vi "Open Excel.vi"(8 "error in (no error)":errorcluster, 9 "Visible":bool, 11 "Excel Interface in":refnum<class "Excel Interface.lvclass">) -> (0 "error out":errorcluster, 3 "Excel Interface out":refnum<class "Excel Interface.lvclass">)   [LabVIEW 2013, in "Excel Interface.lvclass"]
uses:
  Excel Interface.lvclass
  Excel Interface.lvclass/Excel Interface.ctl
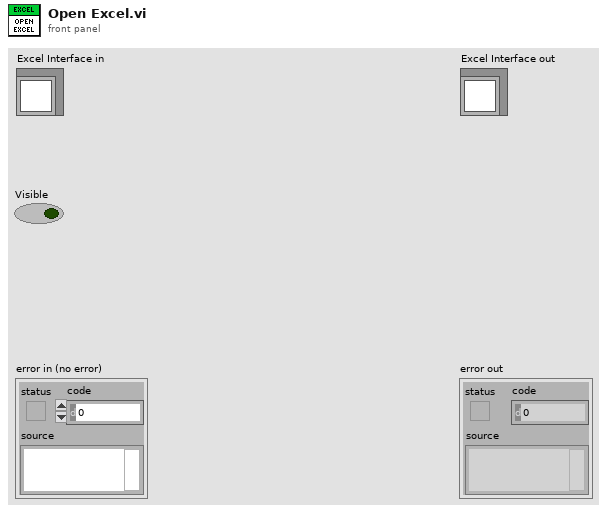
[diagram p1: front panel]
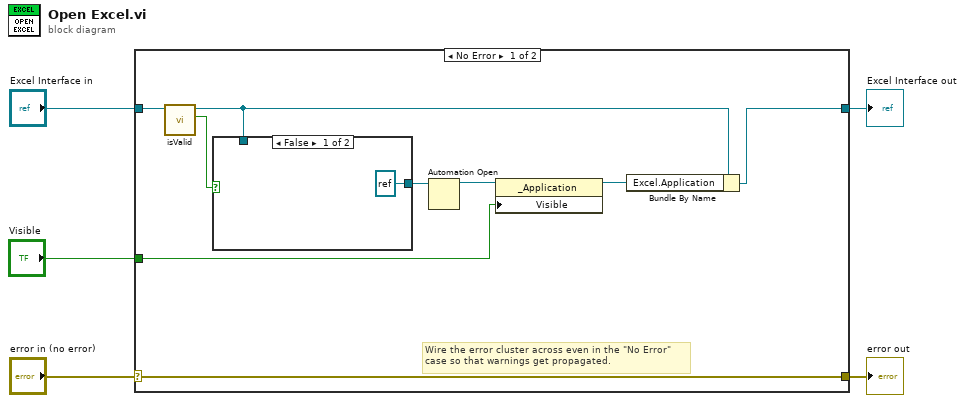
[diagram p0: block diagram]
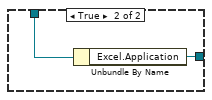
[diagram p2: hidden frame]
diagram:
  n1 = case shown="No Error" "error in (no error)" {
    selector: "error in (no error)" -> [w14 w19]
    tunnel: [w14 w19] -> w4
    tunnel: [w11 w18] -> w2
    tunnel: "Excel Interface in" -> [w9 w18]
    tunnel: "Visible" -> [w12 _]
    frame No Error {
      # "Wire the error cluster across even in the \"No Error\"\ncase so that warnings get propagated."
      n2 = call-dynamic "isValid.vi"("Excel Interface in"=w9) -> ("valid"=w7:bool, "Excel Interface out"=w8:refnum<class "Excel Interface.lvclass">)  [unwired: 8 in, 1 out]
      n3 = case shown="False" w7 {
        tunnel: w8 -> [_ w17]
        tunnel: [refnum<k7> refnum ("Excel.Application") w16] -> w6
        frame False {
        }
        frame True {
          n4 = Unbundle By Name(w17) -> ("Excel.Application"=w16:refnum<k7>)
        }
      }
      n5 = Automation Open(Automation Refnum=w6) -> (Automation Refnum=w13:refnum<k7>)  [unwired: 3 in, 1 out]
      n6 = property class="_Application"(reference=w13, "Visible"=w12) -> (reference out=w10:refnum<k7>)  [unwired: 1 in, 1 out]
      n7 = Bundle By Name(cluster=w8, "Excel.Application"=w10) -> (w11:refnum<class "Excel Interface.lvclass">)
    }
    frame Error {
    }
  }
  "error out" <- w4
  "Excel Interface out" <- w2
